vi "Get ID.vi"(11 "Transceiver Thread in":refnum<class "Plugin Thread.lvclass">) -> (2 "ID":i32, 3 "Transceiver Thread out":refnum<class "Plugin Thread.lvclass">)   [LabVIEW 2017]
uses:
  Thread/Thread.lvclass
  Thread/Plugin/Plugin Thread.lvclass
  C:/Git/DSF/Core/Classes/Thread/Thread.lvclass
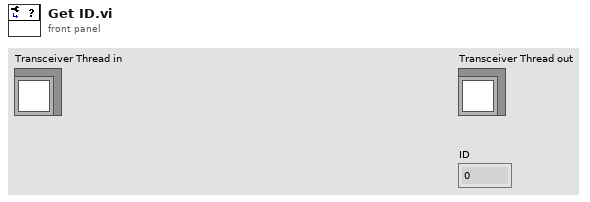
[diagram p1: front panel]
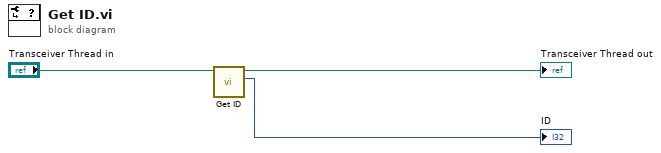
[diagram p0: block diagram]
diagram:
  n1 = call "Get ID.vi"("Thread in"="Transceiver Thread in") -> ("ID"=→"ID":i32, "Thread out"=→"Transceiver Thread out":refnum<class "Plugin Thread.lvclass">)  [unwired: 9 in]
